vi "UI_Run.vi"(0 "reference in":refnum<class "GUI.lvclass">, 5 "error in (no error)":errorcluster) -> (14 "reference out":refnum<class "GUI.lvclass">, 19 "error out":errorcluster)   [LabVIEW 2019, in "GUI.lvclass"]
uses:
  GUI.lvclass
  WindowsState.ctl
  GUI.lvclass/GUI.ctl
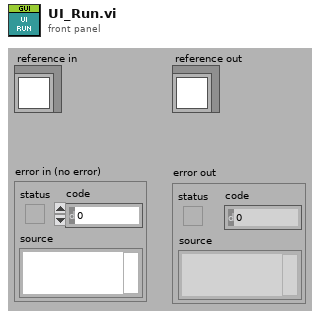
[diagram p1: front panel]
types:
  T1 = typedef "GUI.lvclass/WindowsState.ctl" = enum16{"NotReady", "Ready", "Inserted", "Opened"}
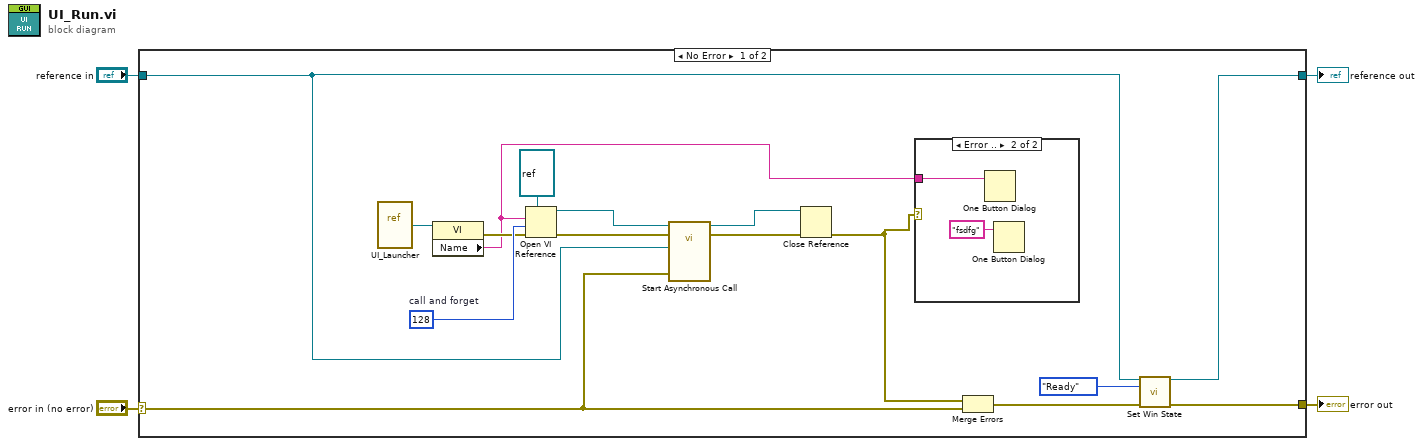
[diagram p0: block diagram]
diagram:
  n1 = case shown="No Error" "error in (no error)" {
    selector: "error in (no error)" -> [w13 w24]
    tunnel: [w10 w24] -> w1
    tunnel: [w9 w23] -> w2
    tunnel: "reference in" -> [w7 w23]
    frame No Error {
      w20 = 128  # call and forget
      n2 = vi-ref "UI_Launcher.vi"() -> (w15:refnum<vi>)
      n3 = property class="VI"(reference=w15) -> (error out=w14:errorcluster, "Name"=w5:string)  [unwired: 1 in, 1 out]
      n4 = Open VI Reference(type specifier VI Refnum (for type only)=refnum<vi> refnum, vi path=w5, options=w20, error in (no error)=w14) -> (vi reference=w12:refnum<vi>, error out=w18:errorcluster)  [unwired: 2 in]
      n5 = call-by-ref "Start Asynchronous Call"(reference=w12, error in=w18, "reference in"=w7, 5:"error in (no error)"=w13) -> (reference out=w16:refnum<vi>, error out=w17:errorcluster)  [unwired: 16 in, 2 out]
      n6 = Close Reference(reference=w16, error in (no error)=w17) -> (error out=w6:errorcluster)
      n7 = case shown="Error .." w6 {
        tunnel: w5 -> [_ w22]
        frame No Error {
        }
        frame Error {
          n8 = One Button Dialog(message=w22) -> ()  [unwired: 1 in, 1 out]
          n9 = One Button Dialog(message="fsdfg") -> ()  [unwired: 1 in, 1 out]
        }
      }
      n10 = Merge Errors(w6, w13) -> (w11:errorcluster)
      n11 = call "Set Win State.vi"("reference in"=w7, "WindowsState"=WindowsState."Ready", "error in (no error)"=w11) -> ("reference out"=w9:refnum<class "GUI.lvclass">, "error out"=w10:errorcluster)  [unwired: 11 in]
    }
    frame Error {
    }
  }
  "error out" <- w1
  "reference out" <- w2
